vi "write test data.vi"(0 "shared memory runtime":refnum<class "Shared Memory runtime.lvclass">, 1 "data allocations":T1, 2 "supported classifications":T4[](array[typedef]), 3 "error in":errorcluster) -> (7 "shared memory runtime out":refnum<class "Shared Memory runtime.lvclass">, 8 "data allocations out":T1, 10 "error out":errorcluster)   [LabVIEW 2013, in "Shared Memory tests.lvlib"]
uses:
  Shared Memory tests.lvlib
  <vilib>/NI/Tag Bus Module Framework/channel/channel classification.ctl
  <vilib>/NI/Tag Bus Module Framework/channel/data tables.ctl
  <vilib>/NI/Tag Bus/dictionary/data dictionary.lvclass
  <vilib>/NI/Tag Bus/dictionary table pair.ctl
  <vilib>/NI/Tag Bus/table/data table.ctl
  module/execution/Shared Memory runtime.lvclass
  module/execution/Shared Memory runtime.lvclass/Shared Memory runtime.ctl
  <vilib>/Analysis/1siggen.llb/Ramp Pattern by Samples.vi
  <vilib>/NI/Tag Bus/table/data polymorphs/write many/write Doubles.vi
  <vilib>/NI/Tag Bus/table/data polymorphs/write many/write Singles.vi
  <vilib>/NI/Tag Bus/table/data polymorphs/write many/write I64s.vi
  <vilib>/NI/Tag Bus/table/data polymorphs/write many/write I32s.vi
  <vilib>/NI/Tag Bus/table/data polymorphs/write many/write I16s.vi
  <vilib>/NI/Tag Bus/table/data polymorphs/write many/write I8s.vi
  <vilib>/NI/Tag Bus/table/data polymorphs/write many/write U64s.vi
  <vilib>/NI/Tag Bus/table/data polymorphs/write many/write U32s.vi
  <vilib>/NI/Tag Bus/table/data polymorphs/write many/write U16s.vi
  <vilib>/NI/Tag Bus/table/data polymorphs/write many/write U8s.vi
  <vilib>/NI/Tag Bus/table/data polymorphs/write many/write Booleans.vi
  module/execution/Read input data.vi
  module/execution/Read processing parameters.vi
  module/execution/Read processing results.vi
  module/execution/Read output data.vi
  <vilib>/NI/Shared Memory Library/Classes/Shared Memory/Shared Memory.lvclass
  <vilib>/NI/Tag Bus/table/data table.lvlib
  <vilib>/Analysis/NI_AALBase.lvlib
  <vilib>/NI/Tag Bus Module Framework/channel/TBM channel.lvclass
  <vilib>/NI/Tag Bus/tag bus.lvlib
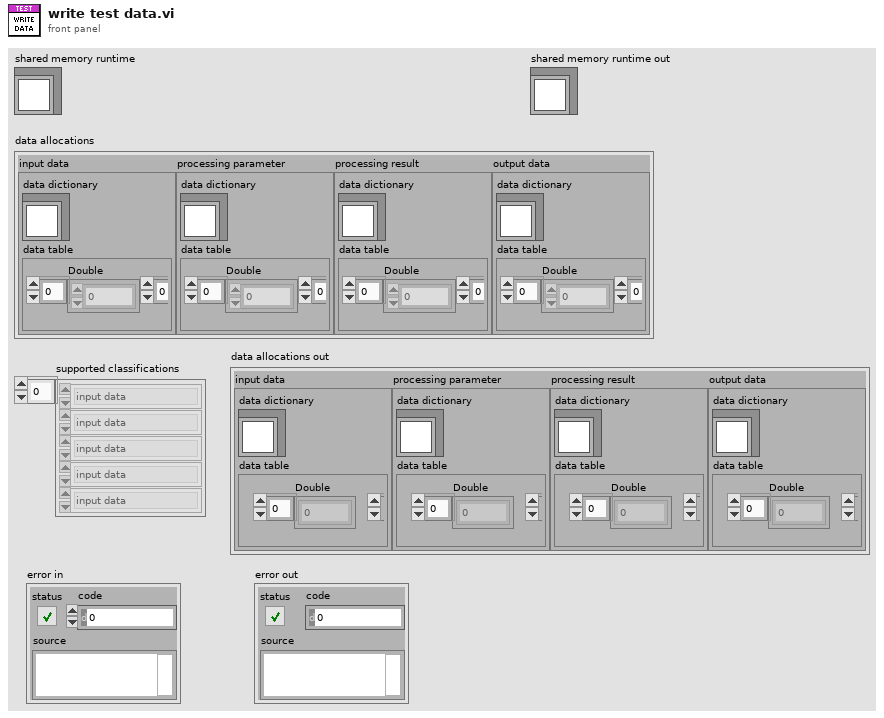
[diagram p1: front panel]
types:
  T1 = typedef "TBM channel.lvclass/data tables.ctl" = cluster{"input data":T2, "processing parameter":T2, "processing result":T2, "output data":T2}
  T2 = typedef "tag bus.lvlib/dictionary table pair.ctl" = cluster{"data dictionary":refnum<class "data dictionary.lvclass">, "data table":T3}
  T3 = typedef "tag bus.lvlib/data table.lvlib/data table.ctl" = cluster{"Double":dbl[], "Single":sgl[], "I64":i64[], "I32":i32[], "I16":i16[], "I8":i8[], "U64":u64[], "U32":u32[], "U16":u16[], "U8":u8[], "Boolean":bool[], "String":string[], "Array of Double":cluster{"DBL Array":dbl[]}[], "Array of Single":cluster{"SGL Array":sgl[]}[], "Array of I64":cluster{"I64 Array":i64[]}[], "Array of I32":cluster{"I32 Array":i32[]}[], "Array of I16":cluster{"I16 Array":i16[]}[], "Array of I8":cluster{"I8 Array":i8[]}[], "Array of U64":cluster{"U64 Array":u64[]}[], "Array of U32":cluster{"U32 Array":u32[]}[], "Array of U16":cluster{"U16 Array":u16[]}[], "Array of U8":cluster{"U8 Array":u8[]}[], "Array of Boolean":cluster{"Boolean Array":bool[]}[], "Array of String":cluster{"String Array":string[]}[]}
  T4 = typedef "TBM channel.lvclass/channel classification.ctl" = enum16{"input data", "output data", "processing parameter", "processing result"}
  T5 = typedef "Shared Memory runtime.lvclass/channel runtime.ctl" = cluster{"channel classification":T4, "data type":T6, "pointer to shared memory":u64, "number of elements":u64, "data dictionary index":cluster{i32[]}, "shared memory":T7}
  T6 = typedef "tag bus.lvlib/tag descriptor.lvclass/Data Type.ctl" = enum16{"Double", "Single", "I64", "I32", "I16", "I8", "U64", "U32", "U16", "U8", "Boolean", "String", "Array of Double", "Array of Single", "Array of I64", "Array of I32", "Array of I16", "Array of I8", "Array of U64", "Array of U32", "Array of U16", "Array of U8", "Array of Boolean", "Array of String"}
  T7 = typedef "Shared Memory.lvlib/Shared Memory.lvclass/reference.ctl" = refnum<data-value>
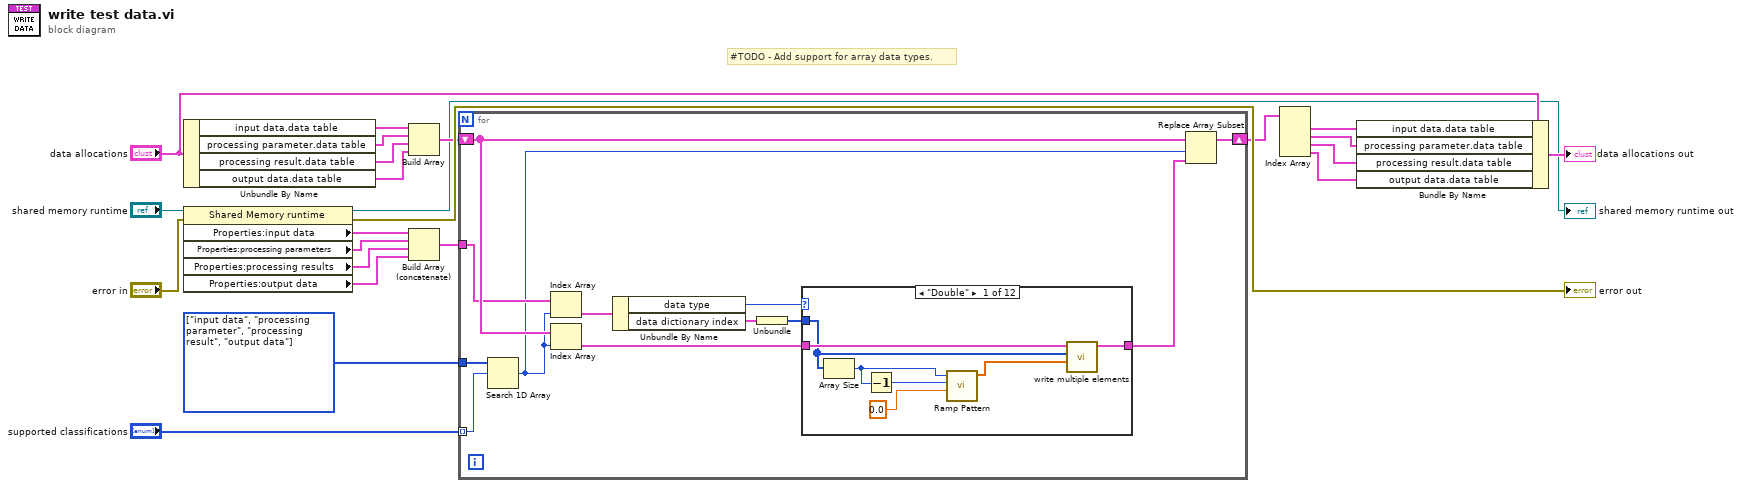
[diagram p0: block diagram]
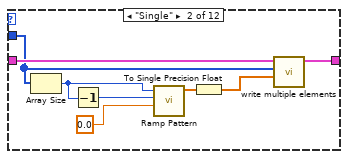
[diagram p2: hidden frame]
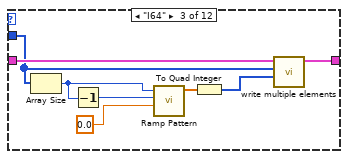
[diagram p3: hidden frame]
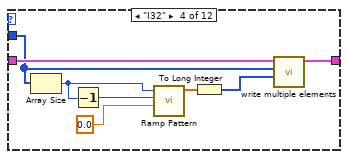
[diagram p4: hidden frame]
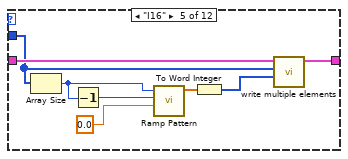
[diagram p5: hidden frame]
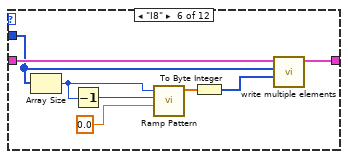
[diagram p6: hidden frame]
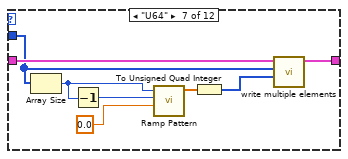
[diagram p7: hidden frame]
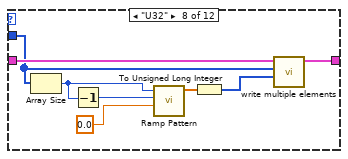
[diagram p8: hidden frame]
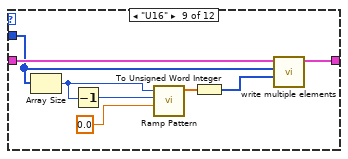
[diagram p9: hidden frame]
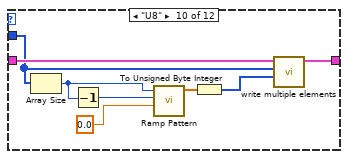
[diagram p10: hidden frame]
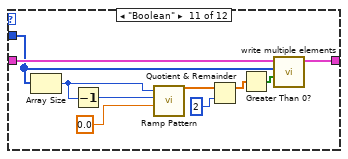
[diagram p11: hidden frame]
diagram:
  w23 = T4[] [enum."input data", enum."processing parameter", enum."processing result", enum."output data"] items=["input data", "output data", "processing parameter", "processing result"] ("supported classifications")
  # "#TODO - Add support for array data types."
  n1 = Unbundle By Name("data allocations") -> ("input data.data table"=w21:T3, "processing parameter.data table"=w18:T3, "processing result.data table"=w19:T3, "output data.data table"=w20:T3)
  n2 = property class="Shared Memory runtime"(reference="shared memory runtime", error in="error in") -> (reference out=→"shared memory runtime out":refnum<class "Shared Memory runtime.lvclass">, error out=→"error out":errorcluster, "Properties:input data"=w14:T5[], "Properties:processing parameters"=w10:T5[], "Properties:processing results"=w11:T5[], "Properties:output data"=w12:T5[])
  n3 = Build Array(w21, w18, w19, w20) -> (w9:T3[])
  n4 = Build Array (concatenate)(w14, w10, w11, w12) -> (w13:T5[])
  n5 = for {
    tunnel: w23 -> [w35]
    tunnel: "supported classifications" -> [w34] mode=indexing
    tunnel: w13 -> [w29]
    shift-right: [w31] -> w7
    shift-left: w9 -> [w32]
    n6 = Search 1D Array(1D array=w35, element=w34) -> (index of element=w28:i32)  [unwired: 1 in]
    n7 = Index Array(array=w29, index=w28) -> (element=w27:T5)
    n8 = Index Array(array=w32, index=w28) -> (element=w33:T3)
    n9 = Unbundle By Name(w27) -> ("data type"=w25:T6, "data dictionary index"=w24:cluster{i32[]})
    n10 = Unbundle(w24) -> (w26:i32[])
    n11 = case shown="\"Double\"" w25 {
      tunnel: w33 -> [w42 w50 w58 w66 w74 w82 w90 w98 w106 w114 w124 w125]
      tunnel: [w40 w48 w56 w64 w72 w80 w88 w96 w104 w112 w122 w125] -> w30
      tunnel: w26 -> [w41 w49 w57 w65 w73 w81 w89 w97 w105 w113 w123 _]
      frame "Double" {
        n12 = Array Size(array=w41) -> (size(s)=w38:i32)
        n13 = Decrement(x=w38) -> (x-1=w37:i32)
        n14 = call-poly <vilib>:"Ramp Pattern.vi"("start"=0.0 ("element"), "end"=w37, "samples"=w38) -> ("Ramp Pattern"=w36:dbl[])  [unwired: 7 in, 1 out]
        n15 = call-poly <vilib>:"write multiple elements.vi"("values"=w36, "indices"=w41, "data table in"=w42) -> ("data table out"=w40:T3)  [unwired: 8 in]
      }
      frame "Single" {
        n16 = Array Size(array=w49) -> (size(s)=w45:i32)
        n17 = Decrement(x=w45) -> (x-1=w44:i32)
        n18 = call-poly <vilib>:"Ramp Pattern.vi"("start"=0.0 ("element"), "end"=w44, "samples"=w45) -> ("Ramp Pattern"=w46:dbl[])  [unwired: 7 in, 1 out]
        n19 = To Single Precision Float(number=w46) -> (single precision float=w43:sgl[])
        n20 = call-poly <vilib>:"write multiple elements.vi"("values"=w43, "indices"=w49, "data table in"=w50) -> ("data table out"=w48:T3)  [unwired: 8 in]
      }
      frame "I64" {
        n21 = Array Size(array=w57) -> (size(s)=w53:i32)
        n22 = Decrement(x=w53) -> (x-1=w52:i32)
        n23 = call-poly <vilib>:"Ramp Pattern.vi"("start"=0.0 ("element"), "end"=w52, "samples"=w53) -> ("Ramp Pattern"=w54:dbl[])  [unwired: 7 in, 1 out]
        n24 = To Quad Integer(1:w54) -> (0:w51:i64[])
        n25 = call-poly <vilib>:"write multiple elements.vi"("values"=w51, "indices"=w57, "data table in"=w58) -> ("data table out"=w56:T3)  [unwired: 8 in]
      }
      frame "I32" {
        n26 = Array Size(array=w65) -> (size(s)=w61:i32)
        n27 = Decrement(x=w61) -> (x-1=w60:i32)
        n28 = call-poly <vilib>:"Ramp Pattern.vi"("start"=0.0 ("element"), "end"=w60, "samples"=w61) -> ("Ramp Pattern"=w62:dbl[])  [unwired: 7 in, 1 out]
        n29 = To Long Integer(number=w62) -> (32bit integer=w59:i32[])
        n30 = call-poly <vilib>:"write multiple elements.vi"("values"=w59, "indices"=w65, "data table in"=w66) -> ("data table out"=w64:T3)  [unwired: 8 in]
      }
      frame "I16" {
        n31 = Array Size(array=w73) -> (size(s)=w69:i32)
        n32 = Decrement(x=w69) -> (x-1=w68:i32)
        n33 = call-poly <vilib>:"Ramp Pattern.vi"("start"=0.0 ("element"), "end"=w68, "samples"=w69) -> ("Ramp Pattern"=w70:dbl[])  [unwired: 7 in, 1 out]
        n34 = To Word Integer(number=w70) -> (16bit integer=w67:i16[])
        n35 = call-poly <vilib>:"write multiple elements.vi"("values"=w67, "indices"=w73, "data table in"=w74) -> ("data table out"=w72:T3)  [unwired: 8 in]
      }
      frame "I8" {
        n36 = Array Size(array=w81) -> (size(s)=w77:i32)
        n37 = Decrement(x=w77) -> (x-1=w76:i32)
        n38 = call-poly <vilib>:"Ramp Pattern.vi"("start"=0.0 ("element"), "end"=w76, "samples"=w77) -> ("Ramp Pattern"=w78:dbl[])  [unwired: 7 in, 1 out]
        n39 = To Byte Integer(number=w78) -> (8bit integer=w75:i8[])
        n40 = call-poly <vilib>:"write multiple elements.vi"("values"=w75, "indices"=w81, "data table in"=w82) -> ("data table out"=w80:T3)  [unwired: 8 in]
      }
      frame "U64" {
        n41 = Array Size(array=w89) -> (size(s)=w85:i32)
        n42 = Decrement(x=w85) -> (x-1=w84:i32)
        n43 = call-poly <vilib>:"Ramp Pattern.vi"("start"=0.0 ("element"), "end"=w84, "samples"=w85) -> ("Ramp Pattern"=w86:dbl[])  [unwired: 7 in, 1 out]
        n44 = To Unsigned Quad Integer(1:w86) -> (0:w83:u64[])
        n45 = call-poly <vilib>:"write multiple elements.vi"("values"=w83, "indices"=w89, "data table in"=w90) -> ("data table out"=w88:T3)  [unwired: 8 in]
      }
      frame "U32" {
        n46 = Array Size(array=w97) -> (size(s)=w93:i32)
        n47 = Decrement(x=w93) -> (x-1=w92:i32)
        n48 = call-poly <vilib>:"Ramp Pattern.vi"("start"=0.0 ("element"), "end"=w92, "samples"=w93) -> ("Ramp Pattern"=w94:dbl[])  [unwired: 7 in, 1 out]
        n49 = To Unsigned Long Integer(number=w94) -> (unsigned 32bit integer=w91:u32[])
        n50 = call-poly <vilib>:"write multiple elements.vi"("values"=w91, "indices"=w97, "data table in"=w98) -> ("data table out"=w96:T3)  [unwired: 8 in]
      }
      frame "U16" {
        n51 = Array Size(array=w105) -> (size(s)=w101:i32)
        n52 = Decrement(x=w101) -> (x-1=w100:i32)
        n53 = call-poly <vilib>:"Ramp Pattern.vi"("start"=0.0 ("element"), "end"=w100, "samples"=w101) -> ("Ramp Pattern"=w102:dbl[])  [unwired: 7 in, 1 out]
        n54 = To Unsigned Word Integer(number=w102) -> (unsigned 16bit integer=w99:u16[])
        n55 = call-poly <vilib>:"write multiple elements.vi"("values"=w99, "indices"=w105, "data table in"=w106) -> ("data table out"=w104:T3)  [unwired: 8 in]
      }
      frame "U8" {
        n56 = Array Size(array=w113) -> (size(s)=w109:i32)
        n57 = Decrement(x=w109) -> (x-1=w108:i32)
        n58 = call-poly <vilib>:"Ramp Pattern.vi"("start"=0.0 ("element"), "end"=w108, "samples"=w109) -> ("Ramp Pattern"=w110:dbl[])  [unwired: 7 in, 1 out]
        n59 = To Unsigned Byte Integer(number=w110) -> (unsigned 8bit integer=w107:u8[])
        n60 = call-poly <vilib>:"write multiple elements.vi"("values"=w107, "indices"=w113, "data table in"=w114) -> ("data table out"=w112:T3)  [unwired: 8 in]
      }
      frame "Boolean" {
        n61 = Array Size(array=w123) -> (size(s)=w120:i32)
        n62 = Decrement(x=w120) -> (x-1=w119:i32)
        n63 = call-poly <vilib>:"Ramp Pattern.vi"("start"=0.0 ("element"), "end"=w119, "samples"=w120) -> ("Ramp Pattern"=w118:dbl[])  [unwired: 7 in, 1 out]
        n64 = Quotient & Remainder(x=w118, y=2) -> (x-y*floor(x/y)=w116:dbl[])  [unwired: 1 out]
        n65 = Greater Than 0?(x=w116) -> (x > 0?=w115:bool[])
        n66 = call-poly <vilib>:"write multiple elements.vi"("values"=w115, "indices"=w123, "data table in"=w124) -> ("data table out"=w122:T3)  [unwired: 8 in]
      }
      frame Default {
      }
    }
    n67 = Replace Array Subset(array=w32, new element=w30, index=w28) -> (w31:T3[])
  }
  n68 = Index Array(array=w7) -> (element #1=w6:T3, element #2=w3:T3, element #3=w4:T3, element #4=w5:T3)  [unwired: 4 in]
  n69 = Bundle By Name(cluster="data allocations", "input data.data table"=w6, "processing parameter.data table"=w3, "processing result.data table"=w4, "output data.data table"=w5) -> (→"data allocations out":T1)
